vi "Estimated Time Required.vi"(1 "Lithography Information":T1(array[cluster])) -> (0 "Estimated Time Required":timestamp format="%<%I:%M:%S>T")   [LabVIEW 2013]
doc: "Calculates the time required to complete lithography."
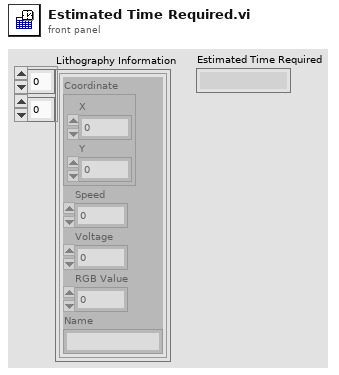
[diagram p1: front panel]
types:
  T1 = cluster{"Coordinate":cluster{"X":dbl, "Y":dbl}, "Speed":dbl, "Voltage":dbl, "RGB Value":i32, "Name":string}[][]
  T2 = cluster{"Coordinate":cluster{"X":dbl, "Y":dbl}, "Speed":dbl, "Voltage":dbl, "RGB Value":i32, "Name":string}
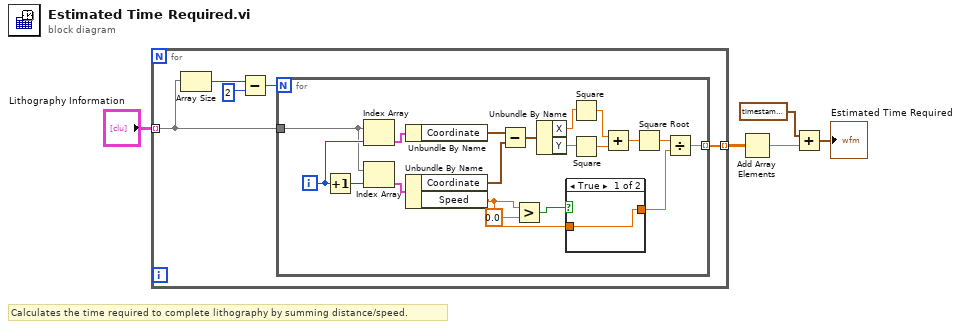
[diagram p0: block diagram]
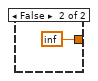
[diagram p2: hidden frame]
diagram:
  # "Calculates the time required to complete lithography by summing distance/speed."
  n1 = for {
    tunnel: "Lithography Information" -> [w10] mode=indexing
    tunnel: [w9] -> w4 mode=indexing
    n2 = Array Size(array=w10) -> (size(s)=w7:i32)
    n3 = Subtract(x=w7, y=2) -> (x-y=w6:i32)
    n4 = for {
      N: w6 -> [_]
      tunnel: w10 -> [w27]
      tunnel: [w15] -> w9 mode=indexing
      i -> [w28]
      n5 = Increment(x=w28) -> (x+1=w29:i32)
      n6 = Index Array(array=w27, index=w28) -> (element=w25:T2)
      n7 = Index Array(array=w27, index=w29) -> (element=w26:T2)
      n8 = Unbundle By Name(w25) -> ("Coordinate"=w23:cluster{"X":dbl, "Y":dbl})
      n9 = Unbundle By Name(w26) -> ("Coordinate"=w24:cluster{"X":dbl, "Y":dbl}, "Speed"=w11:dbl)
      n10 = Subtract(x=w23, y=w24) -> (x-y=w22:cluster{"X":dbl, "Y":dbl})
      n11 = Greater?(x=w11, y=0.0) -> (0:w12:bool)
      n12 = Unbundle By Name(w22) -> ("X"=w21:dbl, "Y"=w20:dbl)
      n13 = case shown="True" w12 {
        tunnel: w11 -> [w30 _]
        tunnel: [w30 inf] -> w14
        frame True {
        }
        frame False {
        }
      }
      n14 = Square(x=w21) -> (x^2=w19:dbl)
      n15 = Square(x=w20) -> (x^2=w18:dbl)
      n16 = Add(x=w19, y=w18) -> (x+y=w17:dbl)
      n17 = Square Root(x=w17) -> (sqrt(x)=w16:dbl)
      n18 = Divide(x=w16, y=w14) -> (x/y=w15:dbl)
    }
  }
  n19 = Add Array Elements(numeric array=w4) -> (sum=w2:dbl)
  n20 = Add(x=timestamp(-68400 s since 1904-01-01), y=w2) -> (x+y=→"Estimated Time Required":timestamp)
